vi "create default alias.vi"(8 "error in":errorcluster, 11 "configuration in":refnum<class "PL_System Configuration.lvclass">) -> (0 "error out":errorcluster, 2 "default alias":string, 3 "configuration out":refnum<class "PL_System Configuration.lvclass">)   [LabVIEW 2013, in "PL_System Configuration.lvclass"]
uses:
  PL_System Configuration.lvclass
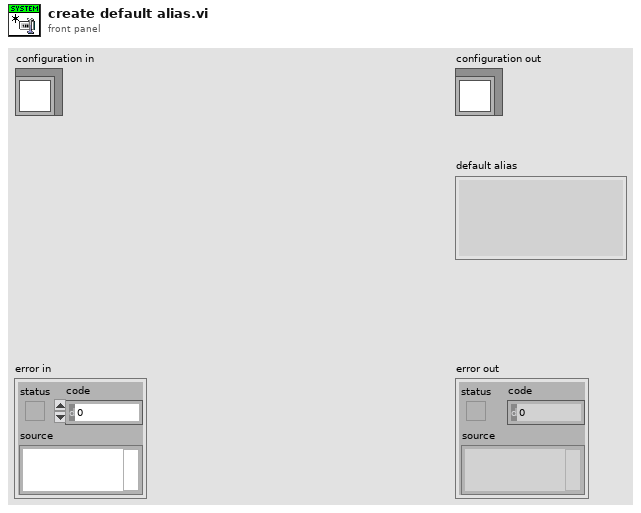
[diagram p1: front panel]
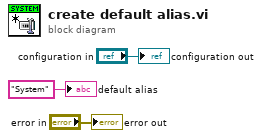
[diagram p0: block diagram]
diagram:
  "error out" <- "error in"
  "configuration out" <- "configuration in"
  "default alias" <- "System" ("default alias")
